vi "test ByRefRead (Unnamed SEQ).vi"(8 "error in (no error)":errorcluster, 11 "TestCase in":refnum<class "Interface Framework Single Object.lvclass">) -> (0 "error out":errorcluster, 3 "TestCase out":refnum<class "Interface Framework Single Object.lvclass">)   [LabVIEW 2009, in "Interface Framework Single Object.lvclass"]
uses:
  Interface Framework Single Object.lvclass
  Numeric Test Object/Interface Implementations/IIntByRef (Unnamed SEQ)/IIntByRef (Unnamed SEQ).lvclass
  Interface Framework Single Object.lvclass/Interface Framework Single Object.ctl
  Numeric Test Object/Numeric Test Object.lvclass
  <vilib>/addons/_JKI Toolkits/VI Tester/TestCase.llb/TestCase.lvclass
  Source/Interfaceable Class/Interfaceable.lvclass
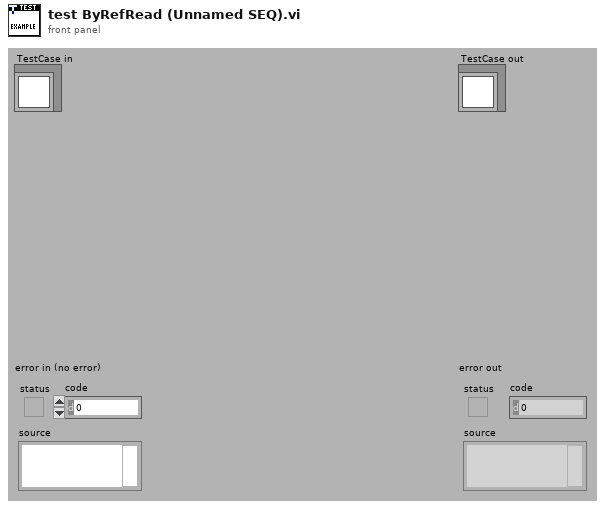
[diagram p1: front panel]
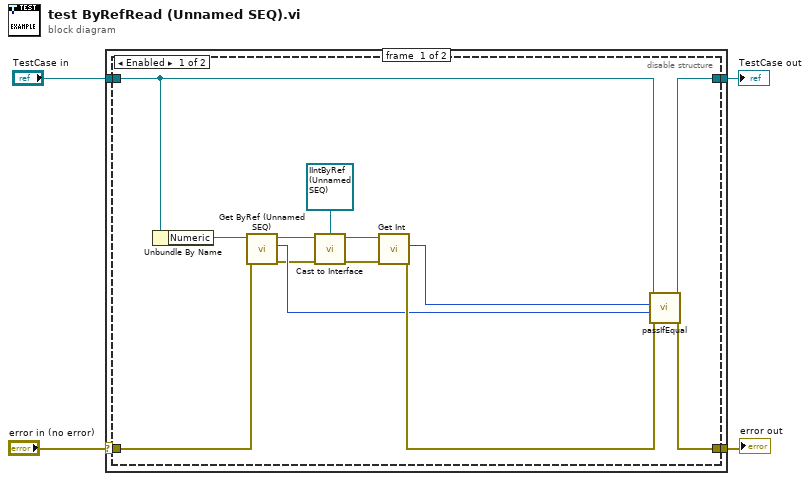
[diagram p0: block diagram]
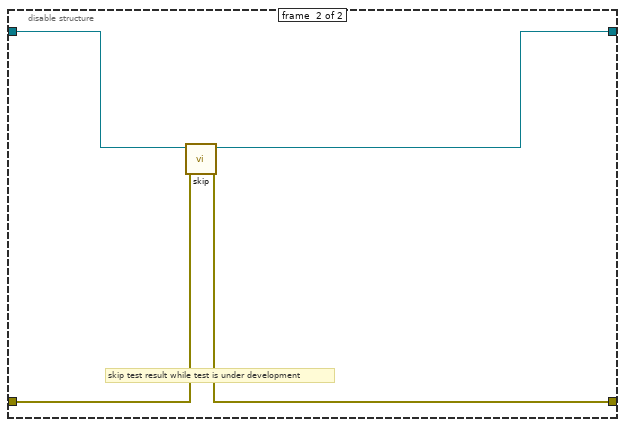
[diagram p2: hidden frame]
diagram:
  n1 = case shown="No Error" "error in (no error)" {
    selector: "error in (no error)" -> [w6 w27]
    tunnel: [w5 w27] -> w3
    tunnel: [w7 w26] -> w1
    tunnel: "TestCase in" -> [w8 w26]
    frame #0 {
      n2 = disable-structure shown="Enabled" {
        disable-tunnel: w8 -> [w19 w25]
        disable-tunnel: [w21 w22] -> w7
        disable-tunnel: w6 -> [w15 w24]
        disable-tunnel: [w20 w23] -> w5
        frame #0 {
          n3 = Unbundle By Name(w19) -> ("Numeric"=w18:refnum<class "Numeric Test Object.lvclass">)
          n4 = call-dynamic "Get ByRef (Unnamed SEQ).vi"("error in (no error)"=w15, "Numeric in"=w18) -> ("error out"=w10:errorcluster, "Int"=w13:i32, "Numeric out"=w17:refnum<class "Numeric Test Object.lvclass">)  [unwired: 7 in]
          n5 = call "Cast to Interface.vi"("Target Interface"=refnum<class "IIntByRef (Unnamed SEQ).lvclass"> refnum ("IIntByRef.lvclass"), "Interfaceable Object"=w17, "error in (no error)"=w10) -> ("Concrete Interface"=w16:refnum<class "IIntByRef (Unnamed SEQ).lvclass">, "error out"=w9:errorcluster)  [unwired: 5 in]
          n6 = call-dynamic "Get Int.vi"("error in (no error)"=w9, "IIntByRef in"=w16) -> ("error out"=w14:errorcluster, "Int"=w12:i32)  [unwired: 7 in, 1 out]
          n7 = call-dynamic "passIfEqual.vi"("error in (no error)"=w14, "y"=w13, "x"=w12, "TestCase in"=w19) -> ("error out"=w20:errorcluster, "TestCase out"=w21:refnum<class "Interface Framework Single Object.lvclass">)  [unwired: 6 in]
        }
        frame #1 {
          # "skip test result while test is under development"
          n8 = call <vilib>:"skip.vi"("error in (no error)"=w24, "TestCase in"=w25) -> ("error out"=w23:errorcluster, "TestCase out"=w22:refnum<class "Interface Framework Single Object.lvclass">)  [unwired: 8 in]
        }
      }
    }
    frame #1 {
    }
  }
  "error out" <- w3
  "TestCase out" <- w1
